vi "test-Signal Change Detector with Period.vi"() -> ()   [LabVIEW 2017]
uses:
  12f2c223-adbf-4fe9-b65d-aec4da49022a.vi
  12f2c223-adbf-4fe9-b65d-aec4da49022a.vi/8970c1ad-ae73-4262-a0e5-fe4d0b54dce3.vi
panel:
  out "Array":u32[](array[numeric])
  in  "stop":bool
  in  "reset":bool
  out "变化过去时间(ms)":u32
  out "周期内信号未变化":bool
  in  "信号":bool
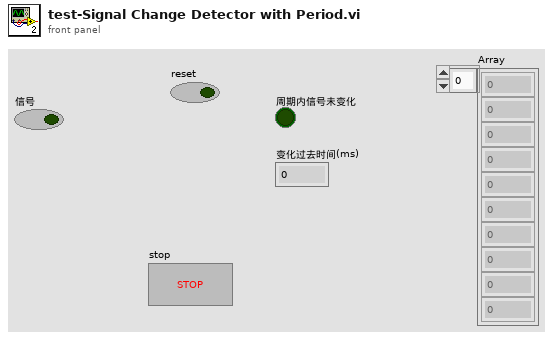
[diagram p1: front panel]
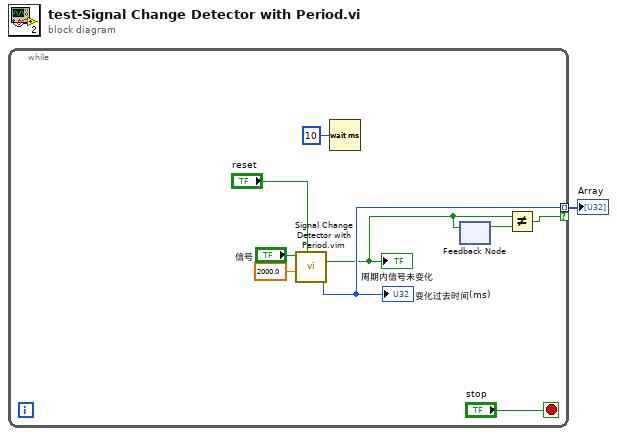
[diagram p0: block diagram]
diagram:
  n1 = while {
    tunnel: [w6] -> w1 mode=indexing if=w4
    stop <- "stop" stop-if-true
    n2 = call "Signal Change Detector with Period.vim"("reset(F)"="reset", "目标时间(ms)"=2000.0 ("计时时长"), "Signal"="信号") -> ("变化过去时间(ms)"=w6:u32, "周期内信号未变化"=w2:bool)  [unwired: 7 in]
    "周期内信号未变化" <- w2
    "变化过去时间(ms)" <- w6
    n3 = Wait (ms)(milliseconds to wait=u32 10) -> ()  [unwired: 1 out]
    n4 = feedback-in #1(w2) -> ()
    n5 = feedback #1() -> (w3:bool)  [unwired: 1 in]
    n6 = Not Equal?(x=w2, y=w3) -> (x != y?=w4:bool)
  }
  "Array" <- w1
